vi "Find Data.vi"(8 "error in (no error)":errorcluster, 10 "Label":string, 11 "data array 1":cluster{"Label":string, "Data":variant}[](array[cluster])) -> (0 "error out":errorcluster, 3 "Value":variant)   [LabVIEW 2017]
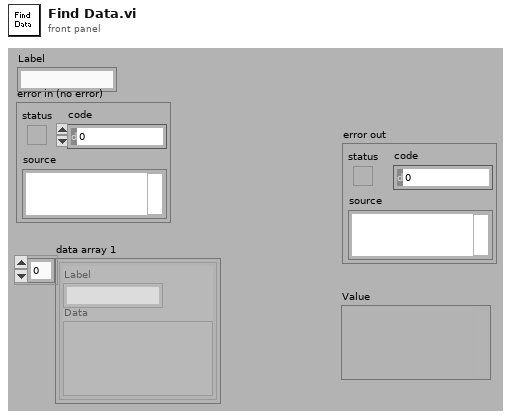
[diagram p1: front panel]
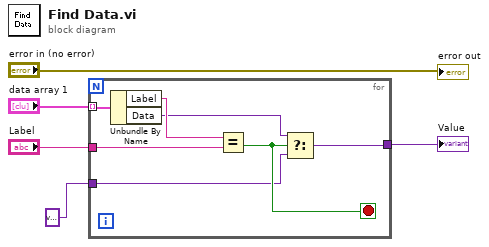
[diagram p0: block diagram]
diagram:
  n1 = for {
    tunnel: "Label" -> [w12]
    tunnel: [w11] -> w3
    tunnel: "data array 1" -> [w9] mode=indexing
    tunnel: variant ("f") -> [w6]
    stop <- w10 stop-if-true
    n2 = Unbundle By Name(w9) -> ("Label"=w8:string, "Data"=w7:variant)
    n3 = Equal?(x=w8, y=w12) -> (x = y?=w10:bool)
    n4 = Select(t=w7, s=w10, f=w6) -> (s? t:f=w11:variant)
  }
  "Value" <- w3
  "error out" <- "error in (no error)"
